vi "find_label_indicies.vi"(8 "error in":errorcluster, 10 "Array":T2[](array[typedef])=[{"Label Array"=["VaporLinePitotdP", "PGinlet-MixingTeePressure", "PGinlet-MixingTeeTemperature"]}, {"Label Array"=["AtmosphericPressure"]}, {"Label Array"=["MegaTankPressure", "MegaTankTemperature", "SeparatorPressure", "SeparatorTemperature", "LiquidInletPressure", "LiquidInletTemperature", "VaporInletPressure", "VaporInletTemperature", "VaporInletPressure", "VaporInletTemperature", "TestSectionPressure", "TSWindow1Temperature", "UpperDevSectionPressure", "UpperDevSectionTemperature", "LowerDevSectionPressure", "UpperDevSectionTemperature"]}, {"Label Array"=["VaporLineDensity", "LiquidLineDensity"]}, {"Label Array"=["VaporInletPressure", "LiquidMassFlow", "VaporMassFlow", "LiquidInletTemperature", "SeparatorTemperature"]}, {"Label Array"=["PGAbsolutePressure", "PGVaporTemperature", "PGLiquidTemperature", "CH4", "CH5", "TSWindow1AbsolutePressure", "TSWindow7AbsolutePressure", "Window1to4dP", "Window1to7dP", "Window1to7FastdP", "VenturidP", "DwyerdP", "CH8", "CH9"]}, {"Label Array"=["MainDiode", "ControlDiode", "TSExteriorTemperature", "TSWindow1AbsolutePressure"]}, {"Label Array"=["VaporMassFlow", "VaporLineDensity", "LiquidMassFlow", "LiquidLineDensity", "CameraVoltage"]}], 11 "haystack":T3[](array[typedef])=[{"Label"="VaporMassFlow", "Offset"=0.0, "Raw"=[2.7002599999999813e-07, -7.932399000000003e-06], "Converted"=[-94.49194574882338, -94.68572460468292], "Average"=-94.58883517675315, "Formula To Output"="(23624.581250*(x-0.004000)+0.000000)*1.000000", "Formula From Output"="(y/1.000000-0.000000)/23624.581250+0.004000"}, {"Label"="VaporLineDensity", "Offset"=0.0, "Raw"=[2.8887519999999912e-06, 1.404330199999999e-05], "Converted"=[-0.499638906, -0.49824458725000004], "Average"=-0.498941746625, "Formula To Output"="(125.000000*(x-0.004000)+0.000000)*1.000000", "Formula From Output"="(y/1.000000-0.000000)/125.000000+0.004000"}, {"Label"="LiquidMassFlow", "Offset"=0.0, "Raw"=[-1.0933037000000001e-05, -7.326225e-06], "Converted"=[-94.75661342091576, -94.67140399776828], "Average"=-94.71400870934201, "Formula To Output"="(23624.581250*(x-0.004000)+0.000000)*1.000000", "Formula From Output"="(y/1.000000-0.000000)/23624.581250+0.004000"}, {"Label"="LiquidLineDensity", "Offset"=0.0, "Raw"=[-1.0776040000000002e-06, 1.2368879e-05], "Converted"=[-0.5001347005, -0.498453890125], "Average"=-0.4992942953125, "Formula To Output"="(125.000000*(x-0.004000)+0.000000)*1.000000", "Formula From Output"="(y/1.000000-0.000000)/125.000000+0.004000"}, {"Label"="VaporInletPressure", "Offset"=0.0, "Raw"=[-4.167609826224644, -3.877966323060606], "Converted"=[-287346.58231237996, -267376.3657629661], "Average"=-277361.47403767303, "Formula To Output"="(10.000000*(x-0.000000)+0.000000)*6894.757290", "Formula From Output"="(y/6894.757290-0.000000)/10.000000+0.000000"}, {"Label"="MegaTankPressure", "Offset"=0.0, "Raw"=[-0.008561255757520144, -0.014964788263964093], "Converted"=[-590.2778054571648, -1031.7858297627288], "Average"=-811.0318176099468, "Formula To Output"="(10.000000*(x-0.000000)+0.000000)*6894.757290", "Formula From Output"="(y/6894.757290-0.000000)/10.000000+0.000000"}, {"Label"="SeparatorPressure", "Offset"=0.0, "Raw"=[0.00867902396488083, 0.008350637685795186], "Converted"=[598.397637519468, 575.7562006028509], "Average"=587.0769190611595, "Formula To Output"="(10.000000*(x-0.000000)+0.000000)*6894.757290", "Formula From Output"="(y/6894.757290-0.000000)/10.000000+0.000000"}, {"Label"="LiquidInletPressure", "Offset"=0.0, "Raw"=[-0.03942956650765626, -0.04731083742526288], "Converted"=[-2718.572911202028, -3261.9674123383606], "Average"=-2990.270161770194, "Formula To Output"="(10.000000*(x-0.000000)+0.000000)*6894.757290", "Formula From Output"="(y/6894.757290-0.000000)/10.000000+0.000000"}, {"Label"="VaporInletTemperature", "Offset"=0.0, "Raw"=[19.193290739375406, 19.193290739375406], "Converted"=[19.193290739375406, 19.193290739375406], "Average"=19.193290739375406, "Formula To Output"="(1.000000*(x-0.000000)+0.000000)*1.000000", "Formula From Output"="(y/1.000000-0.000000)/1.000000+0.000000"}, {"Label"="MegaTankTemperature", "Offset"=0.0, "Raw"=[19.287952509566097, 19.287952509566097], "Converted"=[19.287952509566097, 19.287952509566097], "Average"=19.287952509566097, "Formula To Output"="(1.000000*(x-0.000000)+0.000000)*1.000000", "Formula From Output"="(y/1.000000-0.000000)/1.000000+0.000000"}, {"Label"="LiquidInletTemperature", "Offset"=0.0, "Raw"=[19.3941637547639, 19.3941637547639], "Converted"=[19.3941637547639, 19.3941637547639], "Average"=19.3941637547639, "Formula To Output"="(1.000000*(x-0.000000)+0.000000)*1.000000", "Formula From Output"="(y/1.000000-0.000000)/1.000000+0.000000"}, {"Label"="SeparatorTemperature", "Offset"=0.0, "Raw"=[19.051609358382887, 19.051609358382887], "Converted"=[19.051609358382887, 19.051609358382887], "Average"=19.051609358382887, "Formula To Output"="(1.000000*(x-0.000000)+0.000000)*1.000000", "Formula From Output"="(y/1.000000-0.000000)/1.000000+0.000000"}, {"Label"="LowerDevSectionPressure", "Offset"=0.0, "Raw"=[-0.07817914889993849, -0.08720977206005326], "Converted"=[-5390.2625680384635, -6012.902116702905], "Average"=-5701.582342370684, "Formula To Output"="(10.000000*(x-0.000000)+0.000000)*6894.757290", "Formula From Output"="(y/6894.757290-0.000000)/10.000000+0.000000"}, {"Label"="UpperDevSectionTemperature", "Offset"=0.0, "Raw"=[19.13032655147523, 19.13032655147523], "Converted"=[19.13032655147523, 19.13032655147523], "Average"=19.13032655147523, "Formula To Output"="(1.000000*(x-0.000000)+0.000000)*1.000000", "Formula From Output"="(y/1.000000-0.000000)/1.000000+0.000000"}, {"Label"="UpperDevSectionPressure", "Offset"=0.0, "Raw"=[-0.00084417814944766, -0.0011725644300358679], "Converted"=[-69.84484139955555, -97.01456582381392], "Average"=-83.42970361168474, "Formula To Output"="(12.000000*(x-0.000000)+0.000000)*6894.757290", "Formula From Output"="(y/6894.757290-0.000000)/12.000000+0.000000"}, {"Label"="TestSectionTemperature", "Offset"=0.0, "Raw"=[-55971.21844574473, -55971.21844574473], "Converted"=[-55971.21844574473, -55971.21844574473], "Average"=-55971.21844574473, "Formula To Output"="(1.000000*(x-0.000000)+0.000000)*1.000000", "Formula From Output"="(y/1.000000-0.000000)/1.000000+0.000000"}, {"Label"="TestSectionPressure", "Offset"=0.0, "Raw"=[0.020829316256412263, 0.02033673684046936], "Converted"=[1436.1308010461396, 1402.1686458563765], "Average"=1419.149723451258, "Formula To Output"="(10.000000*(x-0.000000)+0.000000)*6894.757290", "Formula From Output"="(y/6894.757290-0.000000)/10.000000+0.000000"}, {"Label"="DwyerdP", "Offset"=0.0, "Raw"=[0.39676223314155157, 0.3734549473880444], "Converted"=[478.16828696987847, 446.02867129805713], "Average"=462.09847913396777, "Formula To Output"="(0.200000*(x-0.050000)+0.000000)*6894.757290", "Formula From Output"="(y/6894.757290-0.000000)/0.200000+0.050000"}, {"Label"="VenturidP", "Offset"=0.0, "Raw"=[-3.723491999999993e-06, 8.684240000000074e-07], "Converted"=[-628.5233269373349, -627.8078276407022], "Average"=-628.1655772890185, "Formula To Output"="(626.174076*(x-0.004030)+0.000000)*248.840000", "Formula From Output"="(y/248.840000-0.000000)/626.174076+0.004030"}, {"Label"="PGinlet-MixingTeePressure", "Offset"=0.0, "Raw"=[0.04512990065155318, 0.06237017998617466], "Converted"=[3111.59711514272, 4300.272531382898], "Average"=3705.934823262809, "Formula To Output"="(10.000000*(x-0.000000)+0.000000)*6894.757290", "Formula From Output"="(y/6894.757290-0.000000)/10.000000+0.000000"}, {"Label"="PGinlet-MixingTeeTemperature", "Offset"=0.0, "Raw"=[19.168924772592845, 19.168924772592845], "Converted"=[19.168924772592845, 19.168924772592845], "Average"=19.168924772592845, "Formula To Output"="(1.000000*(x-0.000000)+0.000000)*1.000000", "Formula From Output"="(y/1.000000-0.000000)/1.000000+0.000000"}, {"Label"="AtmosphericPressure", "Offset"=0.0, "Raw"=[-0.00018740558843054105, -2.321244820937959e-05], "Converted"=[-43100.30878779386, -43093.23333872818], "Average"=-43096.771063261025, "Formula To Output"="(6.250000*(x-1.000000)+0.000000)*6894.757290", "Formula From Output"="(y/6894.757290-0.000000)/6.250000+1.000000"}, {"Label"="PGAbsolutePressure", "Offset"=0.0, "Raw"=[-0.0006799850091734858, -0.0006799850091734858], "Converted"=[-56.25997918907529, -56.25997918907529], "Average"=-56.25997918907529, "Formula To Output"="(12.000000*(x-0.000000)+0.000000)*6894.757290", "Formula From Output"="(y/6894.757290-0.000000)/12.000000+0.000000"}, {"Label"="PGVaporTemperature", "Offset"=0.0, "Raw"=[18.889761444002122, 18.889761444002122], "Converted"=[18.889761444002122, 18.889761444002122], "Average"=18.889761444002122, "Formula To Output"="(1.000000*(x-0.000000)+0.000000)*1.000000", "Formula From Output"="(y/1.000000-0.000000)/1.000000+0.000000"}, {"Label"="PGLiquidTemperature", "Offset"=0.0, "Raw"=[18.478088702855704, 18.478088702855704], "Converted"=[18.478088702855704, 18.478088702855704], "Average"=18.478088702855704, "Formula To Output"="(1.000000*(x-0.000000)+0.000000)*1.000000", "Formula From Output"="(y/1.000000-0.000000)/1.000000+0.000000"}, {"Label"="Window1to4dP", "Offset"=0.0, "Raw"=[-3.400481000000004e-06, -1.4333390000000037e-06], "Converted"=[-1245.25771961505, -1244.6458400959502], "Average"=-1244.9517798555003, "Formula To Output"="(1250.000000*(x-0.004000)+0.000000)*248.840000", "Formula From Output"="(y/248.840000-0.000000)/1250.000000+0.004000"}, {"Label"="Window1to7dP", "Offset"=0.0, "Raw"=[2.4864230000000013e-06, 2.8142270000000015e-06], "Converted"=[-1243.42659812585, -1243.32463469165], "Average"=-1243.37561640875, "Formula To Output"="(1250.000000*(x-0.004000)+0.000000)*248.840000", "Formula From Output"="(y/248.840000-0.000000)/1250.000000+0.004000"}, {"Label"="Window1to7FastdP", "Offset"=0.0, "Raw"=[1.6242499999999627e-07, 6.388610999999996e-06], "Converted"=[-4309.04832485112, -4302.340818396058], "Average"=-4305.69457162359, "Formula To Output"="(156.250000*(x-0.004000)+0.000000)*6894.757290", "Formula From Output"="(y/6894.757290-0.000000)/156.250000+0.004000"}, {"Label"="CameraVoltage", "Offset"=0.0, "Raw"=[9.597385714, 9.598659526], "Converted"=[47.986928569999996, 47.99329763], "Average"=47.9901131, "Formula To Output"="(5.000000*(x-0.000000)+0.000000)*1.000000", "Formula From Output"="(y/1.000000-0.000000)/5.000000+0.000000"}, {"Label"="CH4", "Offset"=0.0, "Raw"=[19.336982984829888, 19.336982984829888], "Converted"=[19.336982984829888, 19.336982984829888], "Average"=19.336982984829888, "Formula To Output"="(1.000000*(x-0.000000)+0.000000)*1.000000", "Formula From Output"="(y/1.000000-0.000000)/1.000000+0.000000"}, {"Label"="CH5", "Offset"=0.0, "Raw"=[19.198896940499033, 19.198896940499033], "Converted"=[19.198896940499033, 19.198896940499033], "Average"=19.198896940499033, "Formula To Output"="(1.000000*(x-0.000000)+0.000000)*1.000000", "Formula From Output"="(y/1.000000-0.000000)/1.000000+0.000000"}, {"Label"="TSWindow1AbsolutePressure", "Offset"=0.0, "Raw"=[-0.02038316194021679, -0.02071154822413569], "Converted"=[-1405.3695438056025, -1428.010981055461], "Average"=-1416.6902624305317, "Formula To Output"="(10.000000*(x-0.000000)+0.000000)*6894.757290", "Formula From Output"="(y/6894.757290-0.000000)/10.000000+0.000000"}, {"Label"="TSWindow7AbsolutePressure", "Offset"=0.0, "Raw"=[-0.026458308202322624, -0.021696707076245717], "Converted"=[-1824.2361335903067, -1495.9352928293972], "Average"=-1660.085713209852, "Formula To Output"="(10.000000*(x-0.000000)+0.000000)*6894.757290", "Formula From Output"="(y/6894.757290-0.000000)/10.000000+0.000000"}, {"Label"="MainDiode", "Offset"=0.0, "Raw"=[10.356905056, 10.356905056], "Converted"=[10.356905056, 10.356905056], "Average"=10.356905056, "Formula To Output"="(1.000000*(x-0.000000)+0.000000)*1.000000", "Formula From Output"="(y/1.000000-0.000000)/1.000000+0.000000"}, {"Label"="ControlDiode", "Offset"=0.0, "Raw"=[10.457560011000002, 10.457560011000002], "Converted"=[10.457560011000002, 10.457560011000002], "Average"=10.457560011000002, "Formula To Output"="(1.000000*(x-0.000000)+0.000000)*1.000000", "Formula From Output"="(y/1.000000-0.000000)/1.000000+0.000000"}, {"Label"="TSExteriorTemperature", "Offset"=0.0, "Raw"=[18.847556805837517, 18.847556805837517], "Converted"=[18.847556805837517, 18.847556805837517], "Average"=18.847556805837517, "Formula To Output"="(1.000000*(x-0.000000)+0.000000)*1.000000", "Formula From Output"="(y/1.000000-0.000000)/1.000000+0.000000"}, {"Label"="DSExteriorTemperature", "Offset"=0.0, "Raw"=[18.850107676728243, 18.850107676728243], "Converted"=[18.850107676728243, 18.850107676728243], "Average"=18.850107676728243, "Formula To Output"="(1.000000*(x-0.000000)+0.000000)*1.000000", "Formula From Output"="(y/1.000000-0.000000)/1.000000+0.000000"}, {"Label"="PostMixingTeeTemperature", "Offset"=0.0, "Raw"=[19.07943250379799, 19.07943250379799], "Converted"=[190.7943250379799, 190.7943250379799], "Average"=190.7943250379799, "Formula To Output"="(10.000000*(x-0.000000)+0.000000)*1.000000", "Formula From Output"="(y/1.000000-0.000000)/10.000000+0.000000"}, {"Label"="CH8", "Offset"=0.0, "Raw"=[19.101941735356554, 19.101941735356554], "Converted"=[19.101941735356554, 19.101941735356554], "Average"=19.101941735356554, "Formula To Output"="(1.000000*(x-0.000000)+0.000000)*1.000000", "Formula From Output"="(y/1.000000-0.000000)/1.000000+0.000000"}, {"Label"="CH9", "Offset"=0.0, "Raw"=[19.064173065428175, 19.064173065428175], "Converted"=[19.064173065428175, 19.064173065428175], "Average"=19.064173065428175, "Formula To Output"="(1.000000*(x-0.000000)+0.000000)*1.000000", "Formula From Output"="(y/1.000000-0.000000)/1.000000+0.000000"}, {"Label"="Power", "Offset"=0.0, "Raw"=[], "Converted"=[], "Average"=0.0, "Formula To Output"="", "Formula From Output"=""}]) -> (0 "error out":errorcluster, 2 "Indicies":T1[](array[typedef])=[{"Index Array"=[-1, 19, 20]}, {"Index Array"=[21]}, {"Index Array"=[5, 9, 6, 11, 7, 10, 4, 8, 4, 8, 16, -1, 14, 13, 12, 13]}, {"Index Array"=[1, 3]}, {"Index Array"=[4, 2, 0, 10, 11]}, {"Index Array"=[22, 23, 24, 29, 30, 31, 32, 25, 26, 27, 18, 17, 38, 39]}, {"Index Array"=[33, 34, 35, 31]}, {"Index Array"=[0, 1, 2, 3, 28]}], 3 "Needles Out":T3[][](array[typedef])=[[{"Label"="", "Offset"=0.0, "Raw"=[], "Converted"=[], "Average"=0.0, "Formula To Output"="", "Formula From Output"=""}, {"Label"="AtmosphericPressure", "Offset"=0.0, "Raw"=[-0.00018740558843054105, -2.321244820937959e-05], "Converted"=[-43100.30878779386, -43093.23333872818], "Average"=-43096.771063261025, "Formula To Output"="(6.250000*(x-1.000000)+0.000000)*6894.757290", "Formula From Output"="(y/6894.757290-0.000000)/6.250000+1.000000"}, {"Label"="MegaTankPressure", "Offset"=0.0, "Raw"=[-0.008561255757520144, -0.014964788263964093], "Converted"=[-590.2778054571648, -1031.7858297627288], "Average"=-811.0318176099468, "Formula To Output"="(10.000000*(x-0.000000)+0.000000)*6894.757290", "Formula From Output"="(y/6894.757290-0.000000)/10.000000+0.000000"}, {"Label"="VaporLineDensity", "Offset"=0.0, "Raw"=[2.8887519999999912e-06, 1.404330199999999e-05], "Converted"=[-0.499638906, -0.49824458725000004], "Average"=-0.498941746625, "Formula To Output"="(125.000000*(x-0.004000)+0.000000)*1.000000", "Formula From Output"="(y/1.000000-0.000000)/125.000000+0.004000"}, {"Label"="VaporInletPressure", "Offset"=0.0, "Raw"=[-4.167609826224644, -3.877966323060606], "Converted"=[-287346.58231237996, -267376.3657629661], "Average"=-277361.47403767303, "Formula To Output"="(10.000000*(x-0.000000)+0.000000)*6894.757290", "Formula From Output"="(y/6894.757290-0.000000)/10.000000+0.000000"}, {"Label"="PGAbsolutePressure", "Offset"=0.0, "Raw"=[-0.0006799850091734858, -0.0006799850091734858], "Converted"=[-56.25997918907529, -56.25997918907529], "Average"=-56.25997918907529, "Formula To Output"="(12.000000*(x-0.000000)+0.000000)*6894.757290", "Formula From Output"="(y/6894.757290-0.000000)/12.000000+0.000000"}, {"Label"="MainDiode", "Offset"=0.0, "Raw"=[10.356905056, 10.356905056], "Converted"=[10.356905056, 10.356905056], "Average"=10.356905056, "Formula To Output"="(1.000000*(x-0.000000)+0.000000)*1.000000", "Formula From Output"="(y/1.000000-0.000000)/1.000000+0.000000"}, {"Label"="VaporMassFlow", "Offset"=0.0, "Raw"=[2.7002599999999813e-07, -7.932399000000003e-06], "Converted"=[-94.49194574882338, -94.68572460468292], "Average"=-94.58883517675315, "Formula To Output"="(23624.581250*(x-0.004000)+0.000000)*1.000000", "Formula From Output"="(y/1.000000-0.000000)/23624.581250+0.004000"}], [{"Label"="PGinlet-MixingTeePressure", "Offset"=0.0, "Raw"=[0.04512990065155318, 0.06237017998617466], "Converted"=[3111.59711514272, 4300.272531382898], "Average"=3705.934823262809, "Formula To Output"="(10.000000*(x-0.000000)+0.000000)*6894.757290", "Formula From Output"="(y/6894.757290-0.000000)/10.000000+0.000000"}, {"Label"="", "Offset"=0.0, "Raw"=[], "Converted"=[], "Average"=0.0, "Formula To Output"="", "Formula From Output"=""}, {"Label"="MegaTankTemperature", "Offset"=0.0, "Raw"=[19.287952509566097, 19.287952509566097], "Converted"=[19.287952509566097, 19.287952509566097], "Average"=19.287952509566097, "Formula To Output"="(1.000000*(x-0.000000)+0.000000)*1.000000", "Formula From Output"="(y/1.000000-0.000000)/1.000000+0.000000"}, {"Label"="LiquidLineDensity", "Offset"=0.0, "Raw"=[-1.0776040000000002e-06, 1.2368879e-05], "Converted"=[-0.5001347005, -0.498453890125], "Average"=-0.4992942953125, "Formula To Output"="(125.000000*(x-0.004000)+0.000000)*1.000000", "Formula From Output"="(y/1.000000-0.000000)/125.000000+0.004000"}, {"Label"="LiquidMassFlow", "Offset"=0.0, "Raw"=[-1.0933037000000001e-05, -7.326225e-06], "Converted"=[-94.75661342091576, -94.67140399776828], "Average"=-94.71400870934201, "Formula To Output"="(23624.581250*(x-0.004000)+0.000000)*1.000000", "Formula From Output"="(y/1.000000-0.000000)/23624.581250+0.004000"}, {"Label"="PGVaporTemperature", "Offset"=0.0, "Raw"=[18.889761444002122, 18.889761444002122], "Converted"=[18.889761444002122, 18.889761444002122], "Average"=18.889761444002122, "Formula To Output"="(1.000000*(x-0.000000)+0.000000)*1.000000", "Formula From Output"="(y/1.000000-0.000000)/1.000000+0.000000"}, {"Label"="ControlDiode", "Offset"=0.0, "Raw"=[10.457560011000002, 10.457560011000002], "Converted"=[10.457560011000002, 10.457560011000002], "Average"=10.457560011000002, "Formula To Output"="(1.000000*(x-0.000000)+0.000000)*1.000000", "Formula From Output"="(y/1.000000-0.000000)/1.000000+0.000000"}, {"Label"="VaporLineDensity", "Offset"=0.0, "Raw"=[2.8887519999999912e-06, 1.404330199999999e-05], "Converted"=[-0.499638906, -0.49824458725000004], "Average"=-0.498941746625, "Formula To Output"="(125.000000*(x-0.004000)+0.000000)*1.000000", "Formula From Output"="(y/1.000000-0.000000)/125.000000+0.004000"}], [{"Label"="PGinlet-MixingTeeTemperature", "Offset"=0.0, "Raw"=[19.168924772592845, 19.168924772592845], "Converted"=[19.168924772592845, 19.168924772592845], "Average"=19.168924772592845, "Formula To Output"="(1.000000*(x-0.000000)+0.000000)*1.000000", "Formula From Output"="(y/1.000000-0.000000)/1.000000+0.000000"}, {"Label"="", "Offset"=0.0, "Raw"=[], "Converted"=[], "Average"=0.0, "Formula To Output"="", "Formula From Output"=""}, {"Label"="SeparatorPressure", "Offset"=0.0, "Raw"=[0.00867902396488083, 0.008350637685795186], "Converted"=[598.397637519468, 575.7562006028509], "Average"=587.0769190611595, "Formula To Output"="(10.000000*(x-0.000000)+0.000000)*6894.757290", "Formula From Output"="(y/6894.757290-0.000000)/10.000000+0.000000"}, {"Label"="", "Offset"=0.0, "Raw"=[], "Converted"=[], "Average"=0.0, "Formula To Output"="", "Formula From Output"=""}, {"Label"="VaporMassFlow", "Offset"=0.0, "Raw"=[2.7002599999999813e-07, -7.932399000000003e-06], "Converted"=[-94.49194574882338, -94.68572460468292], "Average"=-94.58883517675315, "Formula To Output"="(23624.581250*(x-0.004000)+0.000000)*1.000000", "Formula From Output"="(y/1.000000-0.000000)/23624.581250+0.004000"}, {"Label"="PGLiquidTemperature", "Offset"=0.0, "Raw"=[18.478088702855704, 18.478088702855704], "Converted"=[18.478088702855704, 18.478088702855704], "Average"=18.478088702855704, "Formula To Output"="(1.000000*(x-0.000000)+0.000000)*1.000000", "Formula From Output"="(y/1.000000-0.000000)/1.000000+0.000000"}, {"Label"="TSExteriorTemperature", "Offset"=0.0, "Raw"=[18.847556805837517, 18.847556805837517], "Converted"=[18.847556805837517, 18.847556805837517], "Average"=18.847556805837517, "Formula To Output"="(1.000000*(x-0.000000)+0.000000)*1.000000", "Formula From Output"="(y/1.000000-0.000000)/1.000000+0.000000"}, {"Label"="LiquidMassFlow", "Offset"=0.0, "Raw"=[-1.0933037000000001e-05, -7.326225e-06], "Converted"=[-94.75661342091576, -94.67140399776828], "Average"=-94.71400870934201, "Formula To Output"="(23624.581250*(x-0.004000)+0.000000)*1.000000", "Formula From Output"="(y/1.000000-0.000000)/23624.581250+0.004000"}], [{"Label"="", "Offset"=0.0, "Raw"=[], "Converted"=[], "Average"=0.0, "Formula To Output"="", "Formula From Output"=""}, {"Label"="", "Offset"=0.0, "Raw"=[], "Converted"=[], "Average"=0.0, "Formula To Output"="", "Formula From Output"=""}, {"Label"="SeparatorTemperature", "Offset"=0.0, "Raw"=[19.051609358382887, 19.051609358382887], "Converted"=[19.051609358382887, 19.051609358382887], "Average"=19.051609358382887, "Formula To Output"="(1.000000*(x-0.000000)+0.000000)*1.000000", "Formula From Output"="(y/1.000000-0.000000)/1.000000+0.000000"}, {"Label"="", "Offset"=0.0, "Raw"=[], "Converted"=[], "Average"=0.0, "Formula To Output"="", "Formula From Output"=""}, {"Label"="LiquidInletTemperature", "Offset"=0.0, "Raw"=[19.3941637547639, 19.3941637547639], "Converted"=[19.3941637547639, 19.3941637547639], "Average"=19.3941637547639, "Formula To Output"="(1.000000*(x-0.000000)+0.000000)*1.000000", "Formula From Output"="(y/1.000000-0.000000)/1.000000+0.000000"}, {"Label"="CH4", "Offset"=0.0, "Raw"=[19.336982984829888, 19.336982984829888], "Converted"=[19.336982984829888, 19.336982984829888], "Average"=19.336982984829888, "Formula To Output"="(1.000000*(x-0.000000)+0.000000)*1.000000", "Formula From Output"="(y/1.000000-0.000000)/1.000000+0.000000"}, {"Label"="TSWindow1AbsolutePressure", "Offset"=0.0, "Raw"=[-0.02038316194021679, -0.02071154822413569], "Converted"=[-1405.3695438056025, -1428.010981055461], "Average"=-1416.6902624305317, "Formula To Output"="(10.000000*(x-0.000000)+0.000000)*6894.757290", "Formula From Output"="(y/6894.757290-0.000000)/10.000000+0.000000"}, {"Label"="LiquidLineDensity", "Offset"=0.0, "Raw"=[-1.0776040000000002e-06, 1.2368879e-05], "Converted"=[-0.5001347005, -0.498453890125], "Average"=-0.4992942953125, "Formula To Output"="(125.000000*(x-0.004000)+0.000000)*1.000000", "Formula From Output"="(y/1.000000-0.000000)/125.000000+0.004000"}], [{"Label"="", "Offset"=0.0, "Raw"=[], "Converted"=[], "Average"=0.0, "Formula To Output"="", "Formula From Output"=""}, {"Label"="", "Offset"=0.0, "Raw"=[], "Converted"=[], "Average"=0.0, "Formula To Output"="", "Formula From Output"=""}, {"Label"="LiquidInletPressure", "Offset"=0.0, "Raw"=[-0.03942956650765626, -0.04731083742526288], "Converted"=[-2718.572911202028, -3261.9674123383606], "Average"=-2990.270161770194, "Formula To Output"="(10.000000*(x-0.000000)+0.000000)*6894.757290", "Formula From Output"="(y/6894.757290-0.000000)/10.000000+0.000000"}, {"Label"="", "Offset"=0.0, "Raw"=[], "Converted"=[], "Average"=0.0, "Formula To Output"="", "Formula From Output"=""}, {"Label"="SeparatorTemperature", "Offset"=0.0, "Raw"=[19.051609358382887, 19.051609358382887], "Converted"=[19.051609358382887, 19.051609358382887], "Average"=19.051609358382887, "Formula To Output"="(1.000000*(x-0.000000)+0.000000)*1.000000", "Formula From Output"="(y/1.000000-0.000000)/1.000000+0.000000"}, {"Label"="CH5", "Offset"=0.0, "Raw"=[19.198896940499033, 19.198896940499033], "Converted"=[19.198896940499033, 19.198896940499033], "Average"=19.198896940499033, "Formula To Output"="(1.000000*(x-0.000000)+0.000000)*1.000000", "Formula From Output"="(y/1.000000-0.000000)/1.000000+0.000000"}, {"Label"="", "Offset"=0.0, "Raw"=[], "Converted"=[], "Average"=0.0, "Formula To Output"="", "Formula From Output"=""}, {"Label"="CameraVoltage", "Offset"=0.0, "Raw"=[9.597385714, 9.598659526], "Converted"=[47.986928569999996, 47.99329763], "Average"=47.9901131, "Formula To Output"="(5.000000*(x-0.000000)+0.000000)*1.000000", "Formula From Output"="(y/1.000000-0.000000)/5.000000+0.000000"}], [{"Label"="", "Offset"=0.0, "Raw"=[], "Converted"=[], "Average"=0.0, "Formula To Output"="", "Formula From Output"=""}, {"Label"="", "Offset"=0.0, "Raw"=[], "Converted"=[], "Average"=0.0, "Formula To Output"="", "Formula From Output"=""}, {"Label"="LiquidInletTemperature", "Offset"=0.0, "Raw"=[19.3941637547639, 19.3941637547639], "Converted"=[19.3941637547639, 19.3941637547639], "Average"=19.3941637547639, "Formula To Output"="(1.000000*(x-0.000000)+0.000000)*1.000000", "Formula From Output"="(y/1.000000-0.000000)/1.000000+0.000000"}, {"Label"="", "Offset"=0.0, "Raw"=[], "Converted"=[], "Average"=0.0, "Formula To Output"="", "Formula From Output"=""}, {"Label"="", "Offset"=0.0, "Raw"=[], "Converted"=[], "Average"=0.0, "Formula To Output"="", "Formula From Output"=""}, {"Label"="TSWindow1AbsolutePressure", "Offset"=0.0, "Raw"=[-0.02038316194021679, -0.02071154822413569], "Converted"=[-1405.3695438056025, -1428.010981055461], "Average"=-1416.6902624305317, "Formula To Output"="(10.000000*(x-0.000000)+0.000000)*6894.757290", "Formula From Output"="(y/6894.757290-0.000000)/10.000000+0.000000"}, {"Label"="", "Offset"=0.0, "Raw"=[], "Converted"=[], "Average"=0.0, "Formula To Output"="", "Formula From Output"=""}, {"Label"="", "Offset"=0.0, "Raw"=[], "Converted"=[], "Average"=0.0, "Formula To Output"="", "Formula From Output"=""}], [{"Label"="", "Offset"=0.0, "Raw"=[], "Converted"=[], "Average"=0.0, "Formula To Output"="", "Formula From Output"=""}, {"Label"="", "Offset"=0.0, "Raw"=[], "Converted"=[], "Average"=0.0, "Formula To Output"="", "Formula From Output"=""}, {"Label"="VaporInletPressure", "Offset"=0.0, "Raw"=[-4.167609826224644, -3.877966323060606], "Converted"=[-287346.58231237996, -267376.3657629661], "Average"=-277361.47403767303, "Formula To Output"="(10.000000*(x-0.000000)+0.000000)*6894.757290", "Formula From Output"="(y/6894.757290-0.000000)/10.000000+0.000000"}, {"Label"="", "Offset"=0.0, "Raw"=[], "Converted"=[], "Average"=0.0, "Formula To Output"="", "Formula From Output"=""}, {"Label"="", "Offset"=0.0, "Raw"=[], "Converted"=[], "Average"=0.0, "Formula To Output"="", "Formula From Output"=""}, {"Label"="TSWindow7AbsolutePressure", "Offset"=0.0, "Raw"=[-0.026458308202322624, -0.021696707076245717], "Converted"=[-1824.2361335903067, -1495.9352928293972], "Average"=-1660.085713209852, "Formula To Output"="(10.000000*(x-0.000000)+0.000000)*6894.757290", "Formula From Output"="(y/6894.757290-0.000000)/10.000000+0.000000"}, {"Label"="", "Offset"=0.0, "Raw"=[], "Converted"=[], "Average"=0.0, "Formula To Output"="", "Formula From Output"=""}, {"Label"="", "Offset"=0.0, "Raw"=[], "Converted"=[], "Average"=0.0, "Formula To Output"="", "Formula From Output"=""}], [{"Label"="", "Offset"=0.0, "Raw"=[], "Converted"=[], "Average"=0.0, "Formula To Output"="", "Formula From Output"=""}, {"Label"="", "Offset"=0.0, "Raw"=[], "Converted"=[], "Average"=0.0, "Formula To Output"="", "Formula From Output"=""}, {"Label"="VaporInletTemperature", "Offset"=0.0, "Raw"=[19.193290739375406, 19.193290739375406], "Converted"=[19.193290739375406, 19.193290739375406], "Average"=19.193290739375406, "Formula To Output"="(1.000000*(x-0.000000)+0.000000)*1.000000", "Formula From Output"="(y/1.000000-0.000000)/1.000000+0.000000"}, {"Label"="", "Offset"=0.0, "Raw"=[], "Converted"=[], "Average"=0.0, "Formula To Output"="", "Formula From Output"=""}, {"Label"="", "Offset"=0.0, "Raw"=[], "Converted"=[], "Average"=0.0, "Formula To Output"="", "Formula From Output"=""}, {"Label"="Window1to4dP", "Offset"=0.0, "Raw"=[-3.400481000000004e-06, -1.4333390000000037e-06], "Converted"=[-1245.25771961505, -1244.6458400959502], "Average"=-1244.9517798555003, "Formula To Output"="(1250.000000*(x-0.004000)+0.000000)*248.840000", "Formula From Output"="(y/248.840000-0.000000)/1250.000000+0.004000"}, {"Label"="", "Offset"=0.0, "Raw"=[], "Converted"=[], "Average"=0.0, "Formula To Output"="", "Formula From Output"=""}, {"Label"="", "Offset"=0.0, "Raw"=[], "Converted"=[], "Average"=0.0, "Formula To Output"="", "Formula From Output"=""}], [{"Label"="", "Offset"=0.0, "Raw"=[], "Converted"=[], "Average"=0.0, "Formula To Output"="", "Formula From Output"=""}, {"Label"="", "Offset"=0.0, "Raw"=[], "Converted"=[], "Average"=0.0, "Formula To Output"="", "Formula From Output"=""}, {"Label"="VaporInletPressure", "Offset"=0.0, "Raw"=[-4.167609826224644, -3.877966323060606], "Converted"=[-287346.58231237996, -267376.3657629661], "Average"=-277361.47403767303, "Formula To Output"="(10.000000*(x-0.000000)+0.000000)*6894.757290", "Formula From Output"="(y/6894.757290-0.000000)/10.000000+0.000000"}, {"Label"="", "Offset"=0.0, "Raw"=[], "Converted"=[], "Average"=0.0, "Formula To Output"="", "Formula From Output"=""}, {"Label"="", "Offset"=0.0, "Raw"=[], "Converted"=[], "Average"=0.0, "Formula To Output"="", "Formula From Output"=""}, {"Label"="Window1to7dP", "Offset"=0.0, "Raw"=[2.4864230000000013e-06, 2.8142270000000015e-06], "Converted"=[-1243.42659812585, -1243.32463469165], "Average"=-1243.37561640875, "Formula To Output"="(1250.000000*(x-0.004000)+0.000000)*248.840000", "Formula From Output"="(y/248.840000-0.000000)/1250.000000+0.004000"}, {"Label"="", "Offset"=0.0, "Raw"=[], "Converted"=[], "Average"=0.0, "Formula To Output"="", "Formula From Output"=""}, {"Label"="", "Offset"=0.0, "Raw"=[], "Converted"=[], "Average"=0.0, "Formula To Output"="", "Formula From Output"=""}], [{"Label"="", "Offset"=0.0, "Raw"=[], "Converted"=[], "Average"=0.0, "Formula To Output"="", "Formula From Output"=""}, {"Label"="", "Offset"=0.0, "Raw"=[], "Converted"=[], "Average"=0.0, "Formula To Output"="", "Formula From Output"=""}, {"Label"="VaporInletTemperature", "Offset"=0.0, "Raw"=[19.193290739375406, 19.193290739375406], "Converted"=[19.193290739375406, 19.193290739375406], "Average"=19.193290739375406, "Formula To Output"="(1.000000*(x-0.000000)+0.000000)*1.000000", "Formula From Output"="(y/1.000000-0.000000)/1.000000+0.000000"}, {"Label"="", "Offset"=0.0, "Raw"=[], "Converted"=[], "Average"=0.0, "Formula To Output"="", "Formula From Output"=""}, {"Label"="", "Offset"=0.0, "Raw"=[], "Converted"=[], "Average"=0.0, "Formula To Output"="", "Formula From Output"=""}, {"Label"="Window1to7FastdP", "Offset"=0.0, "Raw"=[1.6242499999999627e-07, 6.388610999999996e-06], "Converted"=[-4309.04832485112, -4302.340818396058], "Average"=-4305.69457162359, "Formula To Output"="(156.250000*(x-0.004000)+0.000000)*6894.757290", "Formula From Output"="(y/6894.757290-0.000000)/156.250000+0.004000"}, {"Label"="", "Offset"=0.0, "Raw"=[], "Converted"=[], "Average"=0.0, "Formula To Output"="", "Formula From Output"=""}, {"Label"="", "Offset"=0.0, "Raw"=[], "Converted"=[], "Average"=0.0, "Formula To Output"="", "Formula From Output"=""}], [{"Label"="", "Offset"=0.0, "Raw"=[], "Converted"=[], "Average"=0.0, "Formula To Output"="", "Formula From Output"=""}, {"Label"="", "Offset"=0.0, "Raw"=[], "Converted"=[], "Average"=0.0, "Formula To Output"="", "Formula From Output"=""}, {"Label"="TestSectionPressure", "Offset"=0.0, "Raw"=[0.020829316256412263, 0.02033673684046936], "Converted"=[1436.1308010461396, 1402.1686458563765], "Average"=1419.149723451258, "Formula To Output"="(10.000000*(x-0.000000)+0.000000)*6894.757290", "Formula From Output"="(y/6894.757290-0.000000)/10.000000+0.000000"}, {"Label"="", "Offset"=0.0, "Raw"=[], "Converted"=[], "Average"=0.0, "Formula To Output"="", "Formula From Output"=""}, {"Label"="", "Offset"=0.0, "Raw"=[], "Converted"=[], "Average"=0.0, "Formula To Output"="", "Formula From Output"=""}, {"Label"="VenturidP", "Offset"=0.0, "Raw"=[-3.723491999999993e-06, 8.684240000000074e-07], "Converted"=[-628.5233269373349, -627.8078276407022], "Average"=-628.1655772890185, "Formula To Output"="(626.174076*(x-0.004030)+0.000000)*248.840000", "Formula From Output"="(y/248.840000-0.000000)/626.174076+0.004030"}, {"Label"="", "Offset"=0.0, "Raw"=[], "Converted"=[], "Average"=0.0, "Formula To Output"="", "Formula From Output"=""}, {"Label"="", "Offset"=0.0, "Raw"=[], "Converted"=[], "Average"=0.0, "Formula To Output"="", "Formula From Output"=""}], [{"Label"="", "Offset"=0.0, "Raw"=[], "Converted"=[], "Average"=0.0, "Formula To Output"="", "Formula From Output"=""}, {"Label"="", "Offset"=0.0, "Raw"=[], "Converted"=[], "Average"=0.0, "Formula To Output"="", "Formula From Output"=""}, {"Label"="", "Offset"=0.0, "Raw"=[], "Converted"=[], "Average"=0.0, "Formula To Output"="", "Formula From Output"=""}, {"Label"="", "Offset"=0.0, "Raw"=[], "Converted"=[], "Average"=0.0, "Formula To Output"="", "Formula From Output"=""}, {"Label"="", "Offset"=0.0, "Raw"=[], "Converted"=[], "Average"=0.0, "Formula To Output"="", "Formula From Output"=""}, {"Label"="DwyerdP", "Offset"=0.0, "Raw"=[0.39676223314155157, 0.3734549473880444], "Converted"=[478.16828696987847, 446.02867129805713], "Average"=462.09847913396777, "Formula To Output"="(0.200000*(x-0.050000)+0.000000)*6894.757290", "Formula From Output"="(y/6894.757290-0.000000)/0.200000+0.050000"}, {"Label"="", "Offset"=0.0, "Raw"=[], "Converted"=[], "Average"=0.0, "Formula To Output"="", "Formula From Output"=""}, {"Label"="", "Offset"=0.0, "Raw"=[], "Converted"=[], "Average"=0.0, "Formula To Output"="", "Formula From Output"=""}], [{"Label"="", "Offset"=0.0, "Raw"=[], "Converted"=[], "Average"=0.0, "Formula To Output"="", "Formula From Output"=""}, {"Label"="", "Offset"=0.0, "Raw"=[], "Converted"=[], "Average"=0.0, "Formula To Output"="", "Formula From Output"=""}, {"Label"="UpperDevSectionPressure", "Offset"=0.0, "Raw"=[-0.00084417814944766, -0.0011725644300358679], "Converted"=[-69.84484139955555, -97.01456582381392], "Average"=-83.42970361168474, "Formula To Output"="(12.000000*(x-0.000000)+0.000000)*6894.757290", "Formula From Output"="(y/6894.757290-0.000000)/12.000000+0.000000"}, {"Label"="", "Offset"=0.0, "Raw"=[], "Converted"=[], "Average"=0.0, "Formula To Output"="", "Formula From Output"=""}, {"Label"="", "Offset"=0.0, "Raw"=[], "Converted"=[], "Average"=0.0, "Formula To Output"="", "Formula From Output"=""}, {"Label"="CH8", "Offset"=0.0, "Raw"=[19.101941735356554, 19.101941735356554], "Converted"=[19.101941735356554, 19.101941735356554], "Average"=19.101941735356554, "Formula To Output"="(1.000000*(x-0.000000)+0.000000)*1.000000", "Formula From Output"="(y/1.000000-0.000000)/1.000000+0.000000"}, {"Label"="", "Offset"=0.0, "Raw"=[], "Converted"=[], "Average"=0.0, "Formula To Output"="", "Formula From Output"=""}, {"Label"="", "Offset"=0.0, "Raw"=[], "Converted"=[], "Average"=0.0, "Formula To Output"="", "Formula From Output"=""}], [{"Label"="", "Offset"=0.0, "Raw"=[], "Converted"=[], "Average"=0.0, "Formula To Output"="", "Formula From Output"=""}, {"Label"="", "Offset"=0.0, "Raw"=[], "Converted"=[], "Average"=0.0, "Formula To Output"="", "Formula From Output"=""}, {"Label"="UpperDevSectionTemperature", "Offset"=0.0, "Raw"=[19.13032655147523, 19.13032655147523], "Converted"=[19.13032655147523, 19.13032655147523], "Average"=19.13032655147523, "Formula To Output"="(1.000000*(x-0.000000)+0.000000)*1.000000", "Formula From Output"="(y/1.000000-0.000000)/1.000000+0.000000"}, {"Label"="", "Offset"=0.0, "Raw"=[], "Converted"=[], "Average"=0.0, "Formula To Output"="", "Formula From Output"=""}, {"Label"="", "Offset"=0.0, "Raw"=[], "Converted"=[], "Average"=0.0, "Formula To Output"="", "Formula From Output"=""}, {"Label"="CH9", "Offset"=0.0, "Raw"=[19.064173065428175, 19.064173065428175], "Converted"=[19.064173065428175, 19.064173065428175], "Average"=19.064173065428175, "Formula To Output"="(1.000000*(x-0.000000)+0.000000)*1.000000", "Formula From Output"="(y/1.000000-0.000000)/1.000000+0.000000"}, {"Label"="", "Offset"=0.0, "Raw"=[], "Converted"=[], "Average"=0.0, "Formula To Output"="", "Formula From Output"=""}, {"Label"="", "Offset"=0.0, "Raw"=[], "Converted"=[], "Average"=0.0, "Formula To Output"="", "Formula From Output"=""}], [{"Label"="", "Offset"=0.0, "Raw"=[], "Converted"=[], "Average"=0.0, "Formula To Output"="", "Formula From Output"=""}, {"Label"="", "Offset"=0.0, "Raw"=[], "Converted"=[], "Average"=0.0, "Formula To Output"="", "Formula From Output"=""}, {"Label"="LowerDevSectionPressure", "Offset"=0.0, "Raw"=[-0.07817914889993849, -0.08720977206005326], "Converted"=[-5390.2625680384635, -6012.902116702905], "Average"=-5701.582342370684, "Formula To Output"="(10.000000*(x-0.000000)+0.000000)*6894.757290", "Formula From Output"="(y/6894.757290-0.000000)/10.000000+0.000000"}, {"Label"="", "Offset"=0.0, "Raw"=[], "Converted"=[], "Average"=0.0, "Formula To Output"="", "Formula From Output"=""}, {"Label"="", "Offset"=0.0, "Raw"=[], "Converted"=[], "Average"=0.0, "Formula To Output"="", "Formula From Output"=""}, {"Label"="", "Offset"=0.0, "Raw"=[], "Converted"=[], "Average"=0.0, "Formula To Output"="", "Formula From Output"=""}, {"Label"="", "Offset"=0.0, "Raw"=[], "Converted"=[], "Average"=0.0, "Formula To Output"="", "Formula From Output"=""}, {"Label"="", "Offset"=0.0, "Raw"=[], "Converted"=[], "Average"=0.0, "Formula To Output"="", "Formula From Output"=""}], [{"Label"="", "Offset"=0.0, "Raw"=[], "Converted"=[], "Average"=0.0, "Formula To Output"="", "Formula From Output"=""}, {"Label"="", "Offset"=0.0, "Raw"=[], "Converted"=[], "Average"=0.0, "Formula To Output"="", "Formula From Output"=""}, {"Label"="UpperDevSectionTemperature", "Offset"=0.0, "Raw"=[19.13032655147523, 19.13032655147523], "Converted"=[19.13032655147523, 19.13032655147523], "Average"=19.13032655147523, "Formula To Output"="(1.000000*(x-0.000000)+0.000000)*1.000000", "Formula From Output"="(y/1.000000-0.000000)/1.000000+0.000000"}, {"Label"="", "Offset"=0.0, "Raw"=[], "Converted"=[], "Average"=0.0, "Formula To Output"="", "Formula From Output"=""}, {"Label"="", "Offset"=0.0, "Raw"=[], "Converted"=[], "Average"=0.0, "Formula To Output"="", "Formula From Output"=""}, {"Label"="", "Offset"=0.0, "Raw"=[], "Converted"=[], "Average"=0.0, "Formula To Output"="", "Formula From Output"=""}, {"Label"="", "Offset"=0.0, "Raw"=[], "Converted"=[], "Average"=0.0, "Formula To Output"="", "Formula From Output"=""}, {"Label"="", "Offset"=0.0, "Raw"=[], "Converted"=[], "Average"=0.0, "Formula To Output"="", "Formula From Output"=""}]])   [LabVIEW 2017]
uses:
  index_array_cluster.ctl
  analog_data.ctl
  label_array_cluster.ctl
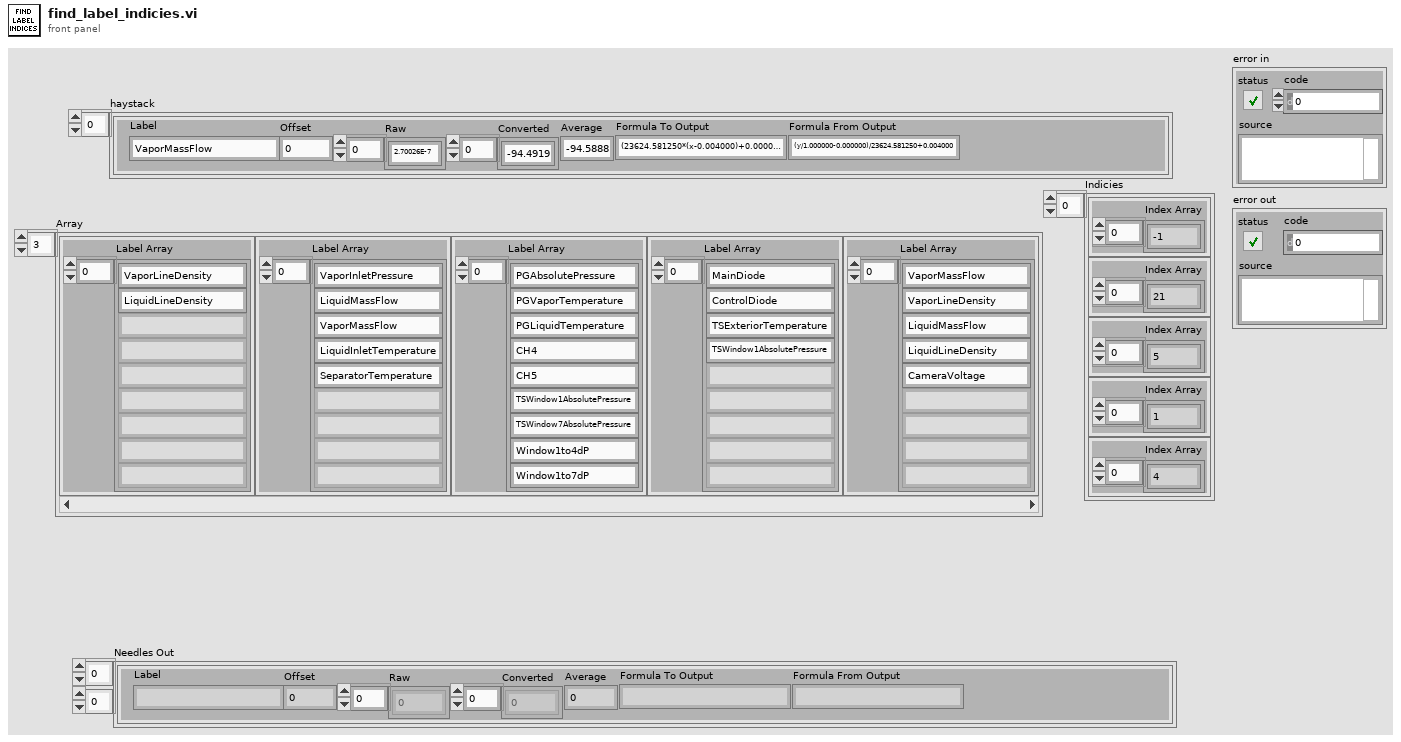
[diagram p1: front panel]
types:
  T1 = typedef "index_array_cluster.ctl" = cluster{"Index Array":i32[]}
  T2 = typedef "label_array_cluster.ctl" = cluster{"Label Array":string[]}
  T3 = typedef "analog_data.ctl" = cluster{"Label":string, "Offset":dbl, "Raw":dbl[], "Converted":dbl[], "Average":dbl, "Formula To Output":string, "Formula From Output":string}
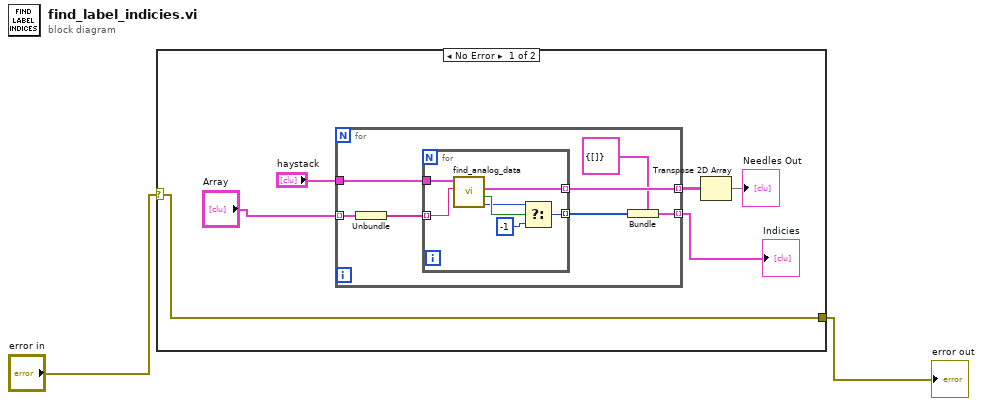
[diagram p0: block diagram]
diagram:
  n1 = case shown="No Error" "error in" {
    selector: "error in" -> [w3 w23]
    tunnel: [w3 w23] -> w1
    frame No Error {
      n2 = for {
        tunnel: "Array" -> [w13] mode=indexing
        tunnel: "haystack" -> [w15]
        tunnel: [w10] -> w4 mode=indexing
        tunnel: [w14] -> w7 mode=indexing
        n3 = Unbundle(w13) -> ("Label Array"=w12:string[])
        n4 = for {
          tunnel: w12 -> [w21] mode=indexing
          tunnel: w15 -> [w22]
          tunnel: [w17] -> w11 mode=indexing
          tunnel: [w16] -> w14 mode=indexing
          n5 = call "find_analog_data.vi"("Needle"=w21, "Haystack"=w22) -> ("Index"=w19:i32, "Found?"=w20:bool, "Needle Out"=w16:T3)  [unwired: 7 in]
          n6 = Select(t=w19, s=w20, f=-1) -> (s? t:f=w17:i32)
        }
        n7 = Bundle(cluster=T1 {"Index Array"=[]} ("Refnum Array Cluster"), "Index Array"=w11) -> (w10:T1)
      }
      "Indicies" <- w4
      n8 = Transpose 2D Array(2D array=w7) -> (transposed array=→"Needles Out":T3[][])
    }
    frame Error {
    }
  }
  "error out" <- w1
